vi "day1-1.vi"() -> ()   [LabVIEW 2021]
uses:
  <vilib>/Utility/file.llb/Read Delimited Spreadsheet (string).vi
panel:
  in  "Example":string="1000\n2000\n3000\n\n4000\n\n5000\n6000\n\n7000\n8000\n9000\n\n10000\n"
  in  "Example":bool
  out "Answer":i32=71934
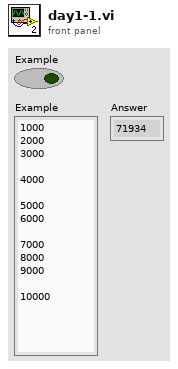
[diagram p1: front panel]
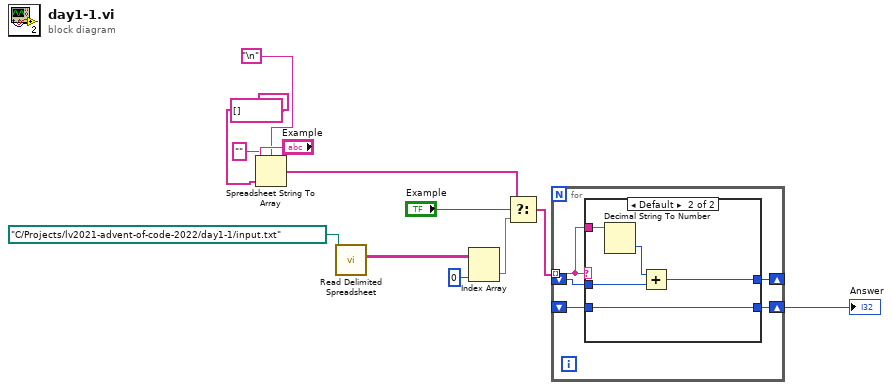
[diagram p0: block diagram]
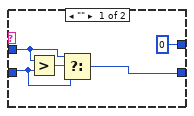
[diagram p2: hidden frame]
diagram:
  n1 = Spreadsheet String To Array(delimiter (Tab)="\n", format string="", spreadsheet string="Example", array type (2D Dbl)=string[] [] ("t")) -> (array=w3:string[])
  n2 = call-poly <vilib>:"Read Delimited Spreadsheet.vi"("file path (dialog if empty)"=path "C:/Projects/lv2021-advent-of-code-2022/day1-1/input.txt") -> ("all rows"=w11:string[][])  [unwired: 9 in, 5 out]
  n3 = Index Array(array=w11, index (col)=0 ("disabled index (col)")) -> (element=w8:string[])  [unwired: 1 in]
  n4 = Select(t=w3, s="Example", f=w8) -> (s? t:f=w7:string[])
  n5 = for {
    tunnel: w7 -> [w15] mode=indexing
    shift-right: [w17] -> _
    shift-left: _ -> [w16]
    shift-right: [w14] -> w9
    shift-left: _ -> [w13]
    n6 = case shown="Default" w15 {
      tunnel: [0 w27] -> w17
      tunnel: w16 -> [w18 w26]
      tunnel: w15 -> [_ w24]
      tunnel: [w19 w23] -> w14
      tunnel: w13 -> [w20 w23]
      frame "" {
        n7 = Greater?(x=w18, y=w20) -> (0:w21:bool)
        n8 = Select(t=w18, s=w21, f=w20) -> (s? t:f=w19:i32)
      }
      frame Default {
        n9 = Decimal String To Number(string=w24) -> (number=w25:i32)  [unwired: 2 in, 1 out]
        n10 = Add(x=w25, y=w26) -> (x+y=w27:i32)
      }
    }
  }
  "Answer" <- w9
